vi "Update FPGABitfile Path (SubVI).vi"(7 "Bitfile Path":path, 8 "error in (no error)":errorcluster, 11 "System Definition path in":path) -> (0 "error out":errorcluster, 3 "System Definition path out":path)   [LabVIEW 2026, in "FPGA Addon Test Class.lvclass"]
uses:
  FPGA Addon Test Class.lvclass
  Addon/Addon System Explorer/FPGA Addon System Explorer.lvlib
  C:/Users/Administrator/Desktop/Jatin/All DNC DLLs/NationalInstruments.VeriStand.SystemDefinitionAPI.dll
  Jatin/All DNC DLLs/NationalInstruments.VeriStand.SystemDefinitionAPI.dll
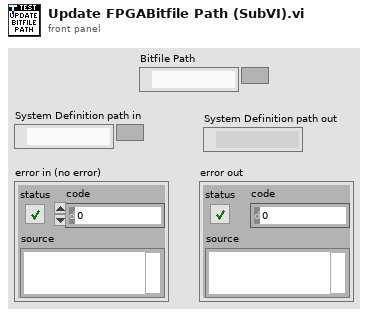
[diagram p1: front panel]
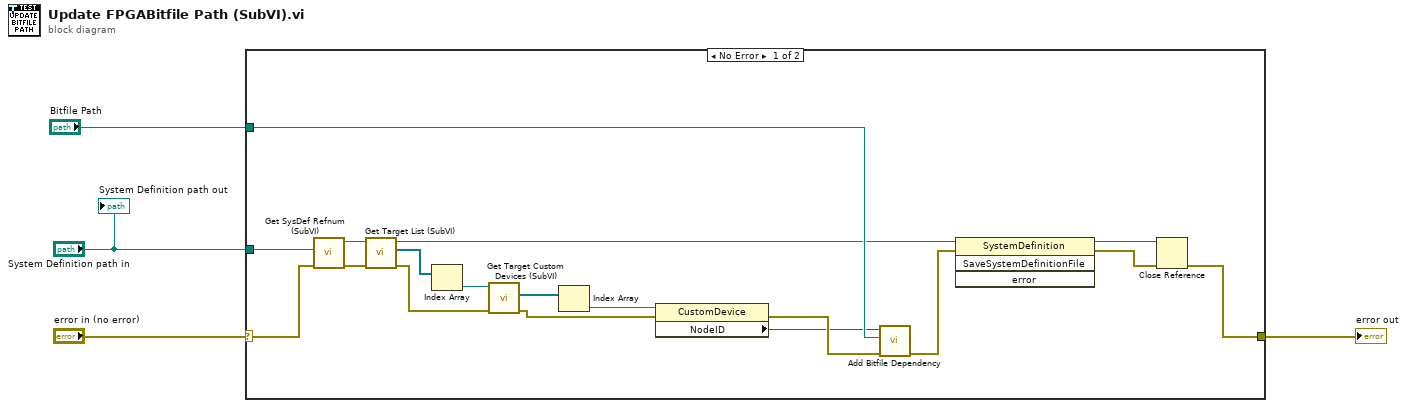
[diagram p0: block diagram]
diagram:
  n1 = case shown="No Error" "error in (no error)" {
    selector: "error in (no error)" -> [w5 w23]
    tunnel: [w22 w23] -> w4
    tunnel: "Bitfile Path" -> [w17 _]
    tunnel: "System Definition path in" -> [w16 _]
    frame No Error {
      n2 = call "Get SysDef Refnum (SubVI).vi"("error in (no error)"=w5, "System Definition path"=w16) -> ("error out"=w6:errorcluster, "NationalInstruments.VeriStand.SystemDefinitionAPI.SystemDefinition"=w7:refnum<k39>)  [unwired: 8 in]
      n3 = call "Get Target List (SubVI).vi"("error in (no error)"=w6, "NationalInstruments.VeriStand.SystemDefinitionAPI.SystemDefinition"=w7) -> ("error out"=w18:errorcluster, "Target List Refnums"=w8:refnum<k39>[], "NationalInstruments.VeriStand.SystemDefinitionAPI.SystemDefinition"=w14:refnum<k39>)  [unwired: 7 in]
      n4 = Index Array(array=w8) -> (element=w9:refnum<k39>)  [unwired: 1 in]
      n5 = call "Get Target Custom Devices (SubVI).vi"("error in (no error)"=w18, "NationalInstruments.VeriStand.SystemDefinitionAPI.Target"=w9) -> ("error out"=w19:errorcluster, "Custom Devices Refnums"=w10:refnum<k39>[])  [unwired: 6 in, 2 out]
      n6 = Index Array(array=w10) -> (element=w11:refnum<k39>)  [unwired: 1 in]
      n7 = property class="CustomDevice"(reference=w11, error in=w19) -> (error out=w13:errorcluster, "NodeID"=w12:u64)  [unwired: 1 out]
      n8 = call "Add Bitfile Dependency.vi"("error in (no error)"=w13, "Path"=w17, "Item Ref in"=w12) -> ("error out"=w15:errorcluster)  [unwired: 6 in, 2 out]
      n9 = invoke class="SystemDefinition" method="SaveSystemDefinitionFile"(reference=w14, error in=w15) -> (reference out=w21:refnum<k39>, error out=w20:errorcluster)  [unwired: 2 in, 2 out]
      n10 = Close Reference(reference=w21, error in (no error)=w20) -> (error out=w22:errorcluster)
    }
    frame Error {
    }
  }
  "error out" <- w4
  "System Definition path out" <- "System Definition path in"
